vi "Inventory-StockTree.vi"(7 "Raw Data From DB Actor":string[][](array[string])=[["1", "tej", "2/28/13", "3/15/2013", "123456987987", "This is a dummy test", "50", "dummy instructions", "unassigned", "2/28/13", "1234556"], ["2", "tej", "2/28/13", "1/25/2013", "123456987987", "This is a dummy test", "50", "dummy instructions", "unassigned", "2/28/13", "1234556"], ["4", "tej", "2/28/13", "3/25/2013", "123456987987", "This is a dummy test", "50", "dummy instructions", "unassigned", "2/28/13", "1234556"], ["6", "tej", "2/28/13", "12/05/2012", "123456987987", "This is a dummy test", "50", "dummy instructions", "unassigned", "2/28/13", "1234556"]], 8 "error in (no error)":errorcluster, 11 "ERP-Inventory in":refnum<class "ERP-Inventory.lvclass">) -> (0 "error out":errorcluster, 3 "ERP-Inventory out":refnum<class "ERP-Inventory.lvclass">)   [LabVIEW 2013, in "ERP-Inventory.lvclass"]
uses:
  ERP-Inventory.lvclass
  ERP-Inventory.lvclass/ERP-Inventory.ctl
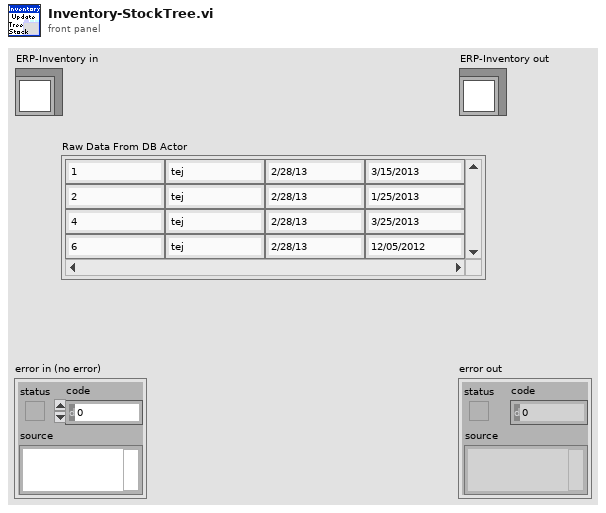
[diagram p1: front panel]
types:
  T1 = typedef "imagedata.ctl" = cluster{"image type":i32, "image depth":i32, "image":u8[], "mask":u8[], "colors":u32[], "Rectangle":cluster{"left":i16, "top":i16, "right":i16, "bottom":i16}}
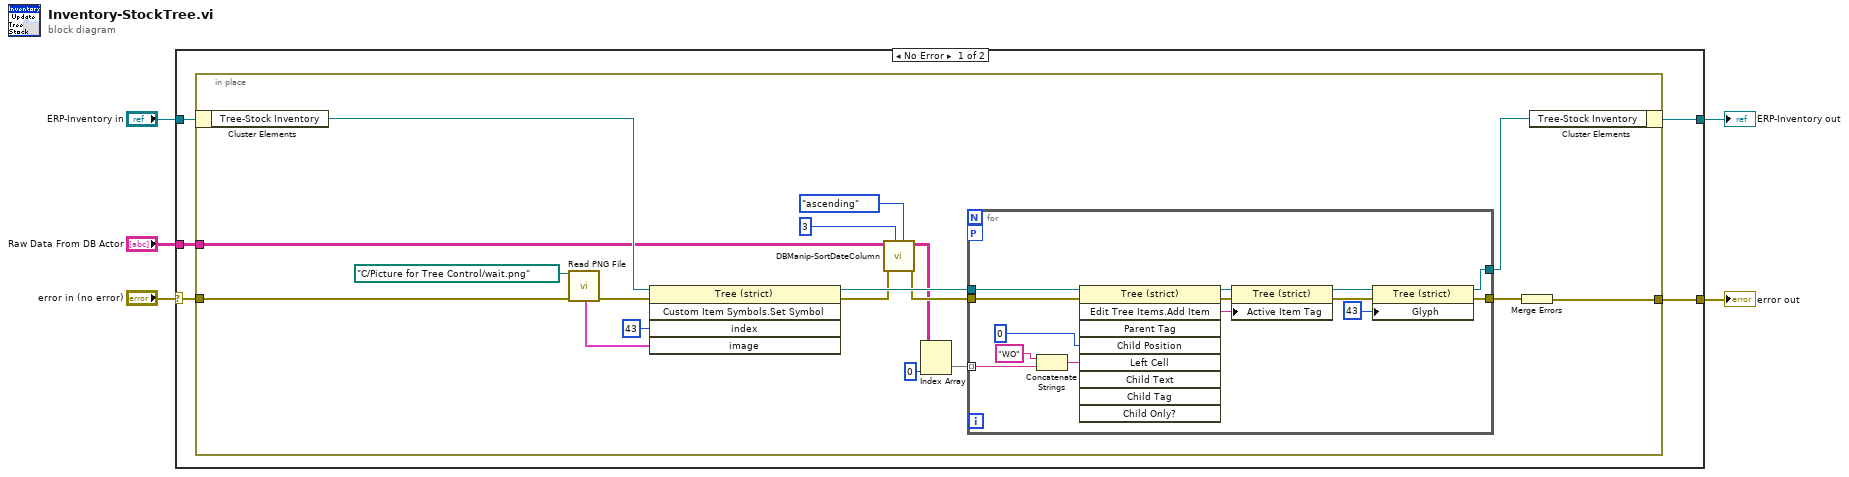
[diagram p0: block diagram]
diagram:
  n1 = case shown="No Error" "error in (no error)" {
    selector: "error in (no error)" -> [w10 w43]
    tunnel: [w7 w44] -> w3
    tunnel: "ERP-Inventory in" -> [w8 w44]
    tunnel: [w9 w43] -> w2
    tunnel: "Raw Data From DB Actor" -> [w6 _]
    frame No Error {
      n2 = in-place {
        in-place-border: w10 -> [w13]
        in-place-border: [w16] -> w9
        in-place-border: w6 -> [w11]
        n3 = in-place-cluster #1(w8) -> ("Tree-Stock Inventory"=w12:refnum<vi>)
        n4 = call <vilib>:"Read PNG File.vi"("error in (no error)"=w13, "path to PNG file"=path "C:/Picture for Tree Control/wait.png") -> ("error out"=w20:errorcluster, "image data"=w27:T1)  [unwired: 7 in, 1 out]
        n5 = invoke class="Tree (strict)" method="Custom Item Symbols.Set Symbol"(reference=w12, error in=w20, "index"=43 ("Index"), "image"=w27) -> (reference out=w28:refnum<vi>, error out=w23:errorcluster)  [unwired: 1 in, 3 out]
        n6 = call "DBManip-SortDateColumn.vi"("Sorting Order"=enum16{"ascending", "descending"}."ascending", "disabled index (col)"=3, "error in"=w23, "DB Table Data"=w11) -> ("error out"=w22:errorcluster, "Sorted Data by Date"=w19:string[][])  [unwired: 6 in]
        n7 = Index Array(array=w19, index (col)=0 ("disabled index (col)")) -> (element=w24:string[])  [unwired: 1 in]
        n8 = for {
          tunnel: w28 -> [w39]
          tunnel: w22 -> [w40]
          tunnel: [w42] -> w15
          tunnel: [w41] -> w17
          tunnel: w24 -> [w29] mode=indexing
          workers-P: _ -> [_]
          n9 = Concatenate Strings("WO" ("string"), w29) -> (w37:string)
          n10 = invoke class="Tree (strict)" method="Edit Tree Items.Add Item"(reference=w39, error in=w40, "Child Position"=0, "Left Cell"=w37) -> (reference out=w33:refnum<vi>, error out=w34:errorcluster, "Edit Tree Items:Add Item"=w36:string)  [unwired: 5 in, 6 out]
          n11 = property class="Tree (strict)"(reference=w33, error in=w34, "Active Item Tag"=w36) -> (reference out=w31:refnum<vi>, error out=w32:errorcluster)
          n12 = property class="Tree (strict)"(reference=w31, error in=w32, "Glyph"=43 ("Active Item:Symbol Index")) -> (reference out=w42:refnum<vi>, error out=w41:errorcluster)
        }
        n13 = Merge Errors(w17) -> (w16:errorcluster)
        n14 = in-place-cluster #1("Tree-Stock Inventory"=w15) -> (w7:refnum<class "ERP-Inventory.lvclass">)
      }
    }
    frame Error {
    }
  }
  "error out" <- w2
  "ERP-Inventory out" <- w3
